vi "Read cell.vi"(8 "error in (no error)":errorcluster, 11 "Speaker Step in":refnum<class "Speaker Step.lvclass">) -> (0 "error out":errorcluster, 2 "cell":u8, 3 "Speaker Step out":refnum<class "Speaker Step.lvclass">)   [LabVIEW 2017, in "Controller.lvlib" / "Speaker Step.lvclass"]
uses:
  Speaker Step.lvclass
  Speaker Step.lvclass/Speaker Step.ctl
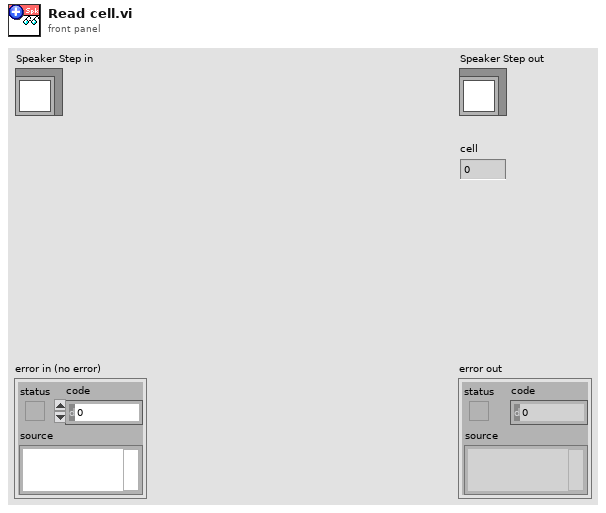
[diagram p1: front panel]
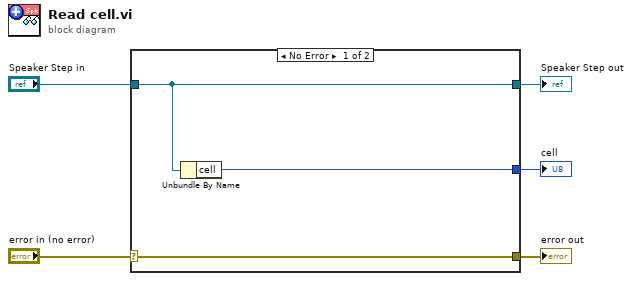
[diagram p0: block diagram]
diagram:
  n1 = case shown="No Error" "error in (no error)" {
    selector: "error in (no error)" -> [w8 w9]
    tunnel: [w8 w9] -> w4
    tunnel: [w7 w10] -> w2
    tunnel: "Speaker Step in" -> [w7 w10]
    tunnel: [w6 _] -> w1
    frame No Error {
      n2 = Unbundle By Name(w7) -> ("cell"=w6:u8)
    }
    frame Error {
    }
  }
  "error out" <- w4
  "Speaker Step out" <- w2
  "cell" <- w1
